vi "Create_JobChild_In_TreeControl.vi"(6 "Child Text":string[](array[string]), 7 "Child Only?":bool, 8 "error in (no error)":errorcluster, 9 "Child Tag Name":string, 10 "Parent Item":string, 11 "TreeControl in":refnum<vi>) -> (0 "error out":errorcluster, 1 "Tag Already Exists?":bool=TRUE, 2 "Edit Tree Items:Add Item 2":string, 3 "TreeControl out":refnum<vi>)   [LabVIEW 2021]
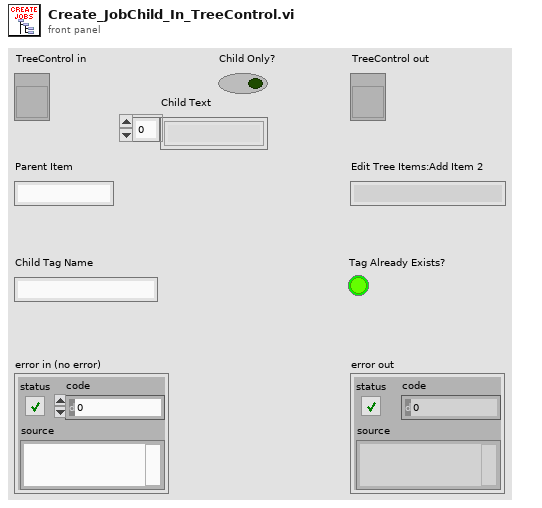
[diagram p1: front panel]
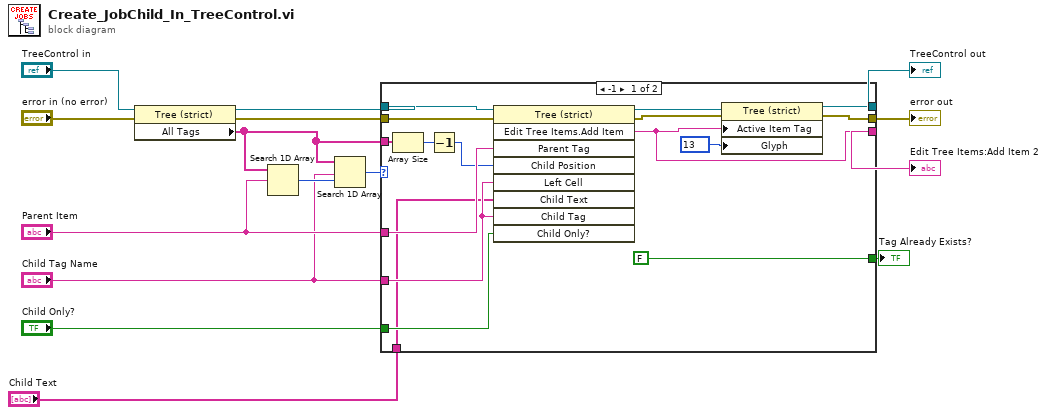
[diagram p0: block diagram]
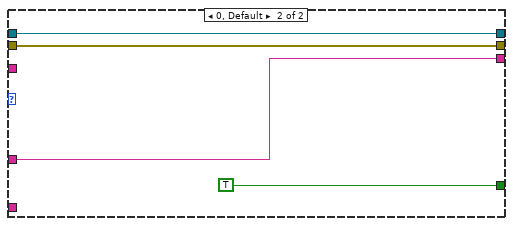
[diagram p2: hidden frame]
diagram:
  n1 = property on="Property Node" class="Tree (strict)"(reference="TreeControl in", error in="error in (no error)") -> (reference out=w10:refnum<vi>, error out=w8:errorcluster, "All Tags"=w3:string[])
  n2 = Search 1D Array(1D array=w3, element="Parent Item") -> (index of element=w6:i32)  [unwired: 1 in]
  n3 = Search 1D Array(1D array=w3, element="Child Tag Name", start index (0)=w6) -> (index of element=w4:i32)
  n4 = case shown="-1" w4 {
    tunnel: "Parent Item" -> [w31 w34]
    tunnel: "Child Only?" -> [w30 _]
    tunnel: [w17 w34] -> w14
    tunnel: [w20 w35] -> w13
    tunnel: w8 -> [w29 w33]
    tunnel: w10 -> [w28 w35]
    tunnel: "Child Tag Name" -> [w27 _]
    tunnel: [w18 w33] -> w12
    tunnel: w3 -> [w26 _]
    tunnel: [FALSE TRUE] -> w2
    tunnel: "Child Text" -> [w16 _]
    frame -1 {
      n5 = Array Size(array=w26) -> (size(s)=w25:i32)
      n6 = Decrement(x=w25) -> (x-1=w24:i32)
      n7 = invoke on="Invoke Node" class="Tree (strict)" method="Edit Tree Items.Add Item"(reference=w28, error in=w29, "Parent Tag"=w31, "Child Position"=w24, "Left Cell"=w27, "Child Text"=w16, "Child Tag"=w27, "Child Only?"=w30) -> (reference out=w21:refnum<vi>, error out=w19:errorcluster, "Edit Tree Items:Add Item"=w17:string)  [unwired: 1 in, 6 out]
      n8 = property class="Tree (strict)"(reference=w21, error in=w19, "Active Item Tag"=w17, "Glyph"=13) -> (reference out=w20:refnum<vi>, error out=w18:errorcluster)
    }
    frame 0, Default {
    }
  }
  "Edit Tree Items:Add Item 2" <- w14
  "TreeControl out" <- w13
  "error out" <- w12
  "Tag Already Exists?" <- w2
